vi "SpectroscopicMeasurementsCtlGFV.vi"(8 "error in (no error)":errorcluster, 10 "Enum":T1=enum."InsertMeasurementScript", 11 "Data in":variant) -> (0 "error out":errorcluster, 3 "Data Out":variant)   [LabVIEW 2017]
doc: "Use this template to build a VI to use as a subVI."
uses:
  SpectroMeasurementCtrlEnum.ctl
  SpectroMeasurementUIMainCluster.ctl
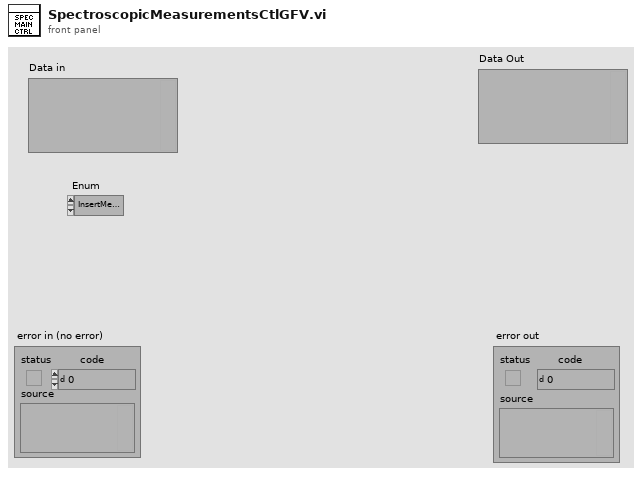
[diagram p1: front panel]
types:
  T1 = typedef "SpectroMeasurementCtrlEnum.ctl" = enum16{"Init", "InsertMeasurementScript", "InsertSetupIndex", "InsertCurrentUserIndex", "GetAllData!"}
  T2 = typedef "SpectroMeasurementUIMainCluster.ctl" = cluster{"idUsers":u32, "idMeas_setup":u32, "idMeas_script":u32}
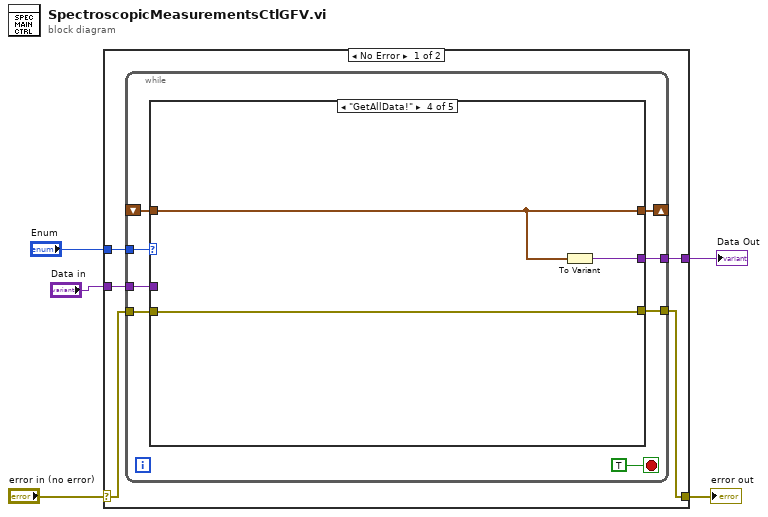
[diagram p0: block diagram]
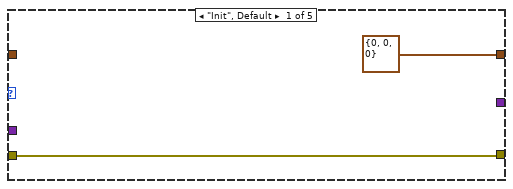
[diagram p2: hidden frame]
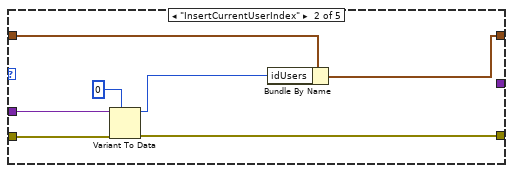
[diagram p3: hidden frame]
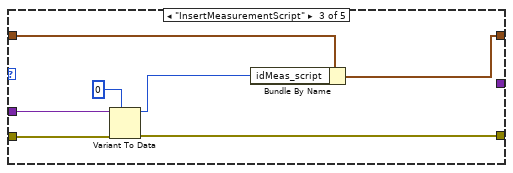
[diagram p4: hidden frame]
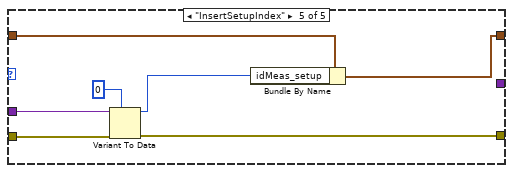
[diagram p5: hidden frame]
diagram:
  n1 = case shown="No Error" "error in (no error)" {
    selector: "error in (no error)" -> [w8 w45]
    tunnel: [w7 w45] -> w4
    tunnel: "Enum" -> [w10 _]
    tunnel: "Data in" -> [w9 _]
    tunnel: [w6 _] -> w1
    frame No Error {
      n2 = while {
        tunnel: w10 -> [w17]
        shift-right: [w16] -> _
        shift-left: _ -> [w15]
        tunnel: w9 -> [w14]
        tunnel: w8 -> [w13]
        tunnel: [w12] -> w7
        tunnel: [w11] -> w6
        stop <- TRUE stop-if-true
        n3 = case shown="\"GetAllData!\"" w17 {
          tunnel: [T2 {"idUsers"=0, "idMeas_setup"=0, "idMeas_script"=0} w26 w33 w36 w43] -> w16
          tunnel: w15 -> [_ w27 w34 w36 w44]
          tunnel: w14 -> [_ w25 w32 _ w42]
          tunnel: w13 -> [w19 w24 w31 w37 w41]
          tunnel: [w19 w23 w30 w37 w40] -> w12
          tunnel: [_ _ _ w35 _] -> w11
          frame "Init", Default {
          }
          frame "InsertCurrentUserIndex" {
            n4 = Variant To Data(error in=w24, type=0 ("element"), Variant=w25) -> (data=w21:i32, error out=w23:errorcluster)
            n5 = Bundle By Name(cluster=w27, "idUsers"=w21) -> (w26:T2)
          }
          frame "InsertMeasurementScript" {
            n6 = Variant To Data(error in=w31, type=0 ("element"), Variant=w32) -> (data=w28:i32, error out=w30:errorcluster)
            n7 = Bundle By Name(cluster=w34, "idMeas_script"=w28) -> (w33:T2)
          }
          frame "GetAllData!" {
            n8 = To Variant(anything=w36) -> (Variant=w35:variant)
          }
          frame "InsertSetupIndex" {
            n9 = Variant To Data(error in=w41, type=0 ("element"), Variant=w42) -> (data=w38:i32, error out=w40:errorcluster)
            n10 = Bundle By Name(cluster=w44, "idMeas_setup"=w38) -> (w43:T2)
          }
        }
      }
    }
    frame Error {
    }
  }
  "error out" <- w4
  "Data Out" <- w1
